vi "UnloadAction.vi"(8 "error in (no error)":errorcluster caption="entrée d'erreur (pas d'erreur)", 11 "Tools In":refnum<class "KlingerMotor.lvclass"> caption="DNL_LabVIEW Object in") -> (0 "error out":errorcluster caption="sortie d'erreur", 3 "Tools Out":refnum<class "KlingerMotor.lvclass"> caption="DNL_LabVIEW Object out")   [LabVIEW 2019, in "KlingerMotor.lvclass"]
uses:
  KlingerMotor.lvclass
  C:/Programmes Labview/Labview 2019/LabscanV1A/DevicesClass/BaseDevice/BaseDevice.lvclass
  BaseDevice/BaseDevice.lvclass
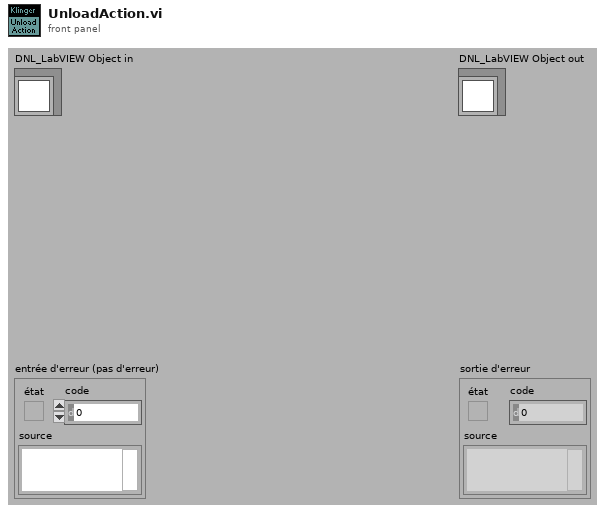
[diagram p1: front panel]
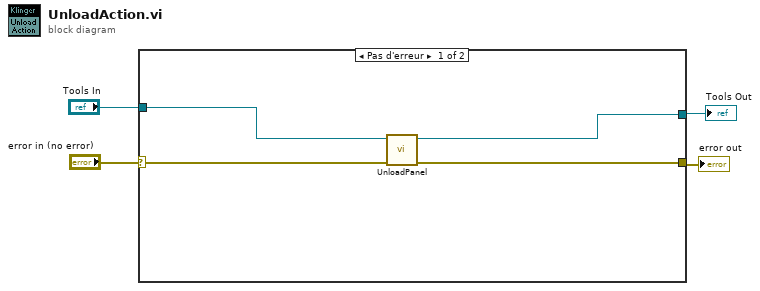
[diagram p0: block diagram]
diagram:
  n1 = case shown="Pas d'erreur" "error in (no error)" {
    selector: "error in (no error)" -> [w6 w9]
    tunnel: [w8 w9] -> w3
    tunnel: [w7 w10] -> w2
    tunnel: "Tools In" -> [w5 w10]
    frame No Error {
      n2 = call "UnloadPanel.vi"("error in (no error)"=w6, "Device en entrée"=w5) -> ("error out"=w8:errorcluster, "Device en sortie"=w7:refnum<class "KlingerMotor.lvclass">)  [unwired: 8 in]
    }
    frame Error {
    }
  }
  "error out" <- w3
  "Tools Out" <- w2
